vi "Match Closing Character.vi"(10 "Open character":string, 11 "JSON":string) -> (1 "offset past match":i32, 2 "rest of JSON":string, 3 "match":string)   [LabVIEW 2015, in "NI_JSON Parsing.lvlib"]
uses:
  NI_JSON Parsing.lvlib
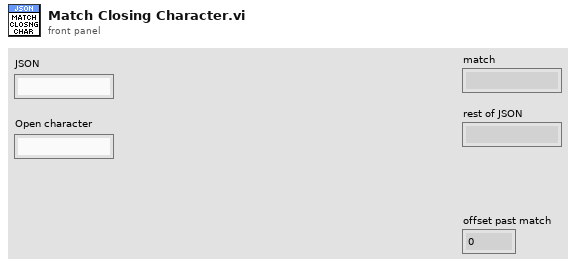
[diagram p1: front panel]
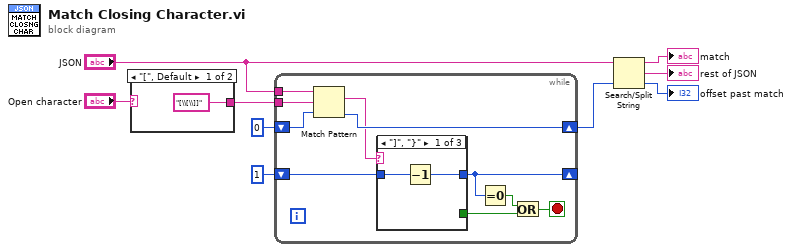
[diagram p0: block diagram]
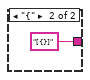
[diagram p2: hidden frame]
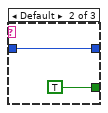
[diagram p3: hidden frame]
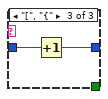
[diagram p4: hidden frame]
diagram:
  n1 = case shown="\"[\", Default" "Open character" {
    tunnel: ["[\\[\\]]" ("regular expression") "[{}]" ("regular expression")] -> w5
    frame "[", Default {
    }
    frame "{" {
    }
  }
  n2 = while {
    tunnel: "JSON" -> [w19]
    shift-right: [w18] -> w4
    shift-left: 0 -> [w20]
    shift-right: [w15] -> _
    shift-left: 1 -> [w17]
    tunnel: w5 -> [w11]
    stop <- w12 stop-if-true
    n3 = Match Pattern(string=w19, regular expression=w11, offset (0)=w20) -> (match substring=w16:string, offset past match=w18:i32)  [unwired: 2 out]
    n4 = case shown="\"]\", \"}\"" w16 {
      tunnel: w17 -> [w22 w23 w26]
      tunnel: [_ TRUE _] -> w14
      tunnel: [w21 w23 w25] -> w15
      frame "]", "}" {
        n5 = Decrement(x=w22) -> (x-1=w21:i32)
      }
      frame Default {
      }
      frame "[", "{" {
        n6 = Increment(x=w26) -> (x+1=w25:i32)
      }
    }
    n7 = Equal To 0?(x=w15) -> (x = 0?=w13:bool)
    n8 = Or(x=w13, y=w14) -> (x .or. y?=w12:bool)
  }
  "offset past match" <- w4
  n9 = Search/Split String(string="JSON", offset (0)=w4) -> (substring before match=→"match":string, match + rest of string=→"rest of JSON":string)  [unwired: 1 in, 1 out]
